vi "Vision Aided Pseudo Code.vi"() -> ()   [LabVIEW 2015]
uses:
  Robot Global Data.vi
panel:
  in  "Movement Speed":dbl
  in  "Turn Speed":dbl
  out "Shoot Wheels":dbl
  out "Right Wheels":dbl
  out "Left Wheels":dbl
  in  "Shoot Button":bool
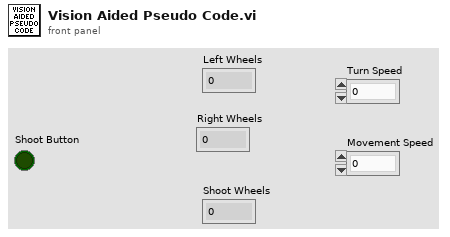
[diagram p1: front panel]
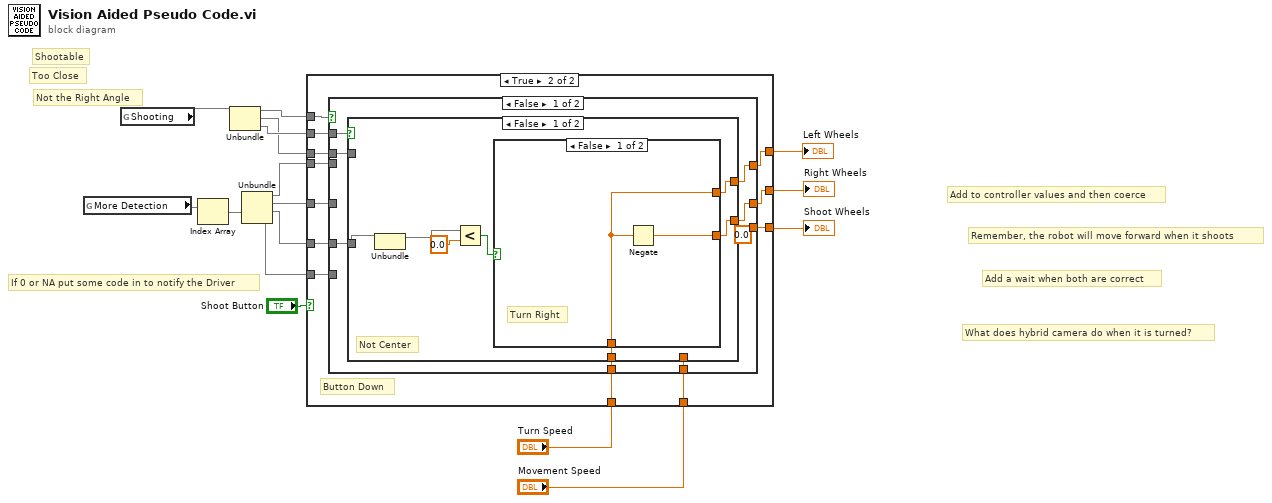
[diagram p0: block diagram]
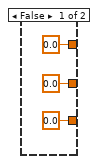
[diagram p2: hidden frame]
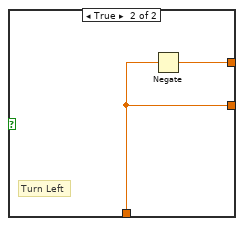
[diagram p3: hidden frame]
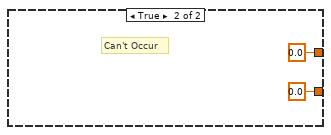
[diagram p5: hidden frame]
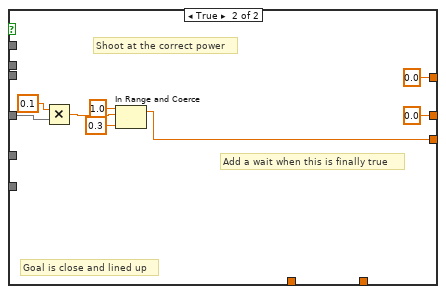
[diagram p6: hidden frame]
diagram:
  # "Not the Right Angle"
  # "Too Close"
  # "Shootable"
  # "What does hybrid camera do when it is turned?"
  # "Add a wait when both are correct"
  # "Remember, the robot will move forward when it shoots"
  # "Add to controller values and then coerce"
  # "If 0 or NA put some code in to notify the Driver"
  n1 = global read "Robot Global Data.vi" "More Detection"() -> (w13)
  n2 = global read "Robot Global Data.vi" "Shooting"() -> (w16)
  n3 = Index Array(array=w13) -> (element=w12)  [unwired: 1 in]
  n4 = Unbundle(w16) -> (w14, w2, w6)
  n5 = Unbundle(w12) -> (w10, w11, w9, w8)
  n6 = case shown="True" "Shoot Button" {
    tunnel: w14 -> [_ w31]
    tunnel: w11 -> [_ w30]
    tunnel: w10 -> [_ w29]
    tunnel: w9 -> [_ w28]
    tunnel: w8 -> [_ w27]
    tunnel: [0.0 ("upper limit") w26] -> w7
    tunnel: w6 -> [_ w25]
    tunnel: "Turn Speed" -> [_ w24]
    tunnel: [0.0 ("Turn Speed") w23] -> w4
    tunnel: [0.0 ("Turn Speed") w22] -> w3
    tunnel: w2 -> [_ w21]
    tunnel: "Movement Speed" -> [_ w20]
    frame False {
    }
    frame True {
      # "Button Down"
      n7 = case shown="False" w31 {
        tunnel: w30 -> [_ w63]
        tunnel: w29 -> [_ _]
        tunnel: w28 -> [w39 _]
        tunnel: w27 -> [_ _]
        tunnel: [0.0 ("upper limit") w60] -> w26
        tunnel: w25 -> [w38 _]
        tunnel: w24 -> [w37 _]
        tunnel: [w36 0.0 ("Turn Speed")] -> w23
        tunnel: [w35 0.0 ("Turn Speed")] -> w22
        tunnel: w21 -> [w33 _]
        tunnel: w20 -> [w32 _]
        frame False {
          n8 = case shown="False" w38 {
            tunnel: w39 -> [w44 _]
            tunnel: w37 -> [w42 _]
            tunnel: [w41 w53] -> w36
            tunnel: [w40 w51] -> w35
            tunnel: w33 -> [_ w54]
            tunnel: w32 -> [_ w52]
            frame False {
              # "Not Center"
              n9 = Unbundle(w44) -> (w43)  [unwired: 1 out]
              n10 = Less?(x=w43, y=0.0) -> (x < y?=w46:bool)
              n11 = case shown="False" w46 {
                tunnel: [w47 w50] -> w41
                tunnel: [w48 w49] -> w40
                tunnel: w42 -> [w47 w49]
                frame False {
                  # "Turn Right"
                  n12 = Negate(x=w47) -> (-x=w48:dbl)
                }
                frame True {
                  # "Turn Left"
                  n13 = Negate(x=w49) -> (-x=w50:dbl)
                }
              }
            }
            frame True {
              # "Center"
              n14 = case shown="False" w54 {
                tunnel: [w55 0.0 ("Movement Speed")] -> w53
                tunnel: w52 -> [w55 _]
                tunnel: [w55 0.0 ("Movement Speed")] -> w51
                frame False {
                  # "Not Close Enough"
                }
                frame True {
                  # "Can't Occur"
                }
              }
            }
          }
        }
        frame True {
          # "Add a wait when this is finally true"
          # "Goal is close and lined up"
          # "Shoot at the correct power"
          n15 = Multiply(x=0.1, y=w63) -> (x*y=w61:dbl)
          n16 = In Range and Coerce(upper limit=1.0, x=w61, lower limit=0.3) -> (coerced(x)=w60:dbl)  [unwired: 1 out]
        }
      }
    }
  }
  "Left Wheels" <- w4
  "Right Wheels" <- w3
  "Shoot Wheels" <- w7
